vi "记录前面板数据.vi"(2 "值班员":string="王伟", 3 "幅值":dbl=6.0 format="%.2f") -> (0 "波形":dbl[](graph)=[0.0, 0.2944060459645081, 0.5881028419773636, 0.8803828467321705, 1.1705419320967696, 1.4578810794195833, 1.741708063526774, 2.0213391203533204, 2.2961005941905386, 2.5653305605816925, 2.8283804209559857, 3.08461646515933, 3.3334213981176135, 3.5741958269546, 3.806359704981873, 4.029353729082111, 4.242640687119285, 4.445706752129754, 4.638062720176421, 4.819245188883869, 4.988817673815271, 5.146371660001632, 5.2915275860901305, 5.42393575874066, 5.543277195067721, 5.649264391098125, 5.741642014393253, 5.820187519167264, 5.884711682419383, 5.935059059788686, 5.971108360033181, 5.992772737231034, 6.0, 5.992772737231034, 5.971108360033181, 5.935059059788686, 5.884711682419383, 5.820187519167264, 5.741642014393253, 5.649264391098125, 5.543277195067721, 5.42393575874066, 5.2915275860901305, 5.146371660001632, 4.988817673815271, 4.81924518888387, 4.638062720176422, 4.445706752129754, 4.242640687119286, 4.029353729082111, 3.8063597049818734, 3.5741958269546004, 3.3334213981176135, 3.0846164651593306, 2.828380420955986, 2.565330560581693, 2.296100594190539, 2.0213391203533204, 1.7417080635267745, 1.4578810794195836, 1.1705419320967698, 0.8803828467321708, 0.588102841977364, 0.2944060459645084, 3.1843017805899265e-16, -0.29440604596450776, -0.5881028419773633, -0.8803828467321702, -1.1705419320967694, -1.4578810794195831, -1.7417080635267739, -2.02133912035332, -2.296100594190538, -2.565330560581692, -2.8283804209559857, -3.08461646515933, -3.333421398117613, -3.5741958269546, -3.8063597049818725, -4.02935372908211, -4.242640687119285, -4.445706752129754, -4.638062720176421, -4.819245188883869, -4.988817673815271, -5.146371660001632, -5.29152758609013, -5.42393575874066, -5.54327719506772, -5.649264391098124, -5.741642014393253, -5.820187519167264, -5.884711682419383, -5.935059059788686, -5.971108360033181, -5.992772737231034, -6.0, -5.992772737231034, -5.971108360033181, -5.935059059788686, -5.884711682419383, -5.8201875191672645, -5.741642014393253, -5.649264391098125, -5.543277195067721, -5.42393575874066, -5.2915275860901305, -5.146371660001632, -4.988817673815272, -4.81924518888387, -4.638062720176422, -4.445706752129755, -4.242640687119286, -4.029353729082111, -3.8063597049818734, -3.5741958269546004, -3.333421398117614, -3.084616465159331, -2.8283804209559866, -2.565330560581693, -2.296100594190539, -2.021339120353321, -1.7417080635267748, -1.457881079419584, -1.1705419320967703, -0.8803828467321712, -0.5881028419773643, -0.2944060459645087], 1 "状态":bool=TRUE)   [LabVIEW 2010]
uses:
  <vilib>/Analysis/NI_AALBase.lvlib
panel:
  # "注意：读者运行此程序应首先改变数据绑定关系，在自己的计算机文件系统中指定数据记录文件的路径与名称。"
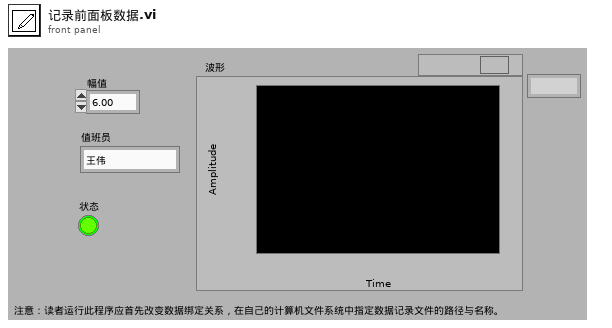
[diagram p1: front panel]
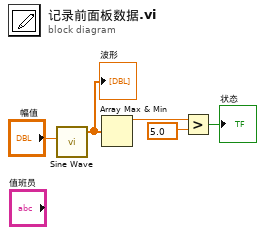
[diagram p0: block diagram]
diagram:
  n1 = call <vilib>:"Sine Wave.vi"("amplitude"="幅值") -> ("sine wave"=w4:dbl[])  [unwired: 4 in, 2 out]
  "波形" <- w4
  n2 = Array Max & Min(array=w4) -> (max value=w3:dbl)  [unwired: 3 out]
  n3 = Greater?(x=w3, y=5.0) -> (0:→"状态":bool)
